vi "Data Save Edit.vi"(10 "Data Path":path, 11 "Project":string) -> (3 "OK?":bool)   [LabVIEW 2020]
uses:
  <vilib>/Utility/miscctls.llb/LVMapReplaceAction.ctl
  <vilib>/Utility/file.llb/Write Delimited Spreadsheet (string).vi
  <vilib>/Utility/config.llb/Read Key (String).vi
  <vilib>/Utility/file.llb/Read Delimited Spreadsheet (string).vi
  <vilib>/Utility/config.llb/NI_LVConfig.lvlib
panel:
  in  "Warning Group Delete":bool
  in  "Warning Group Add":bool
  in  "WarningGroup":i32(listbox)
  in  "Warning Delete":bool
  in  "Warning Export":bool
  in  "Warning Import":bool
  in  "Warning Edit":bool
  in  "Warning List":i32(listbox) caption="报警日志"
  in  "OK":bool
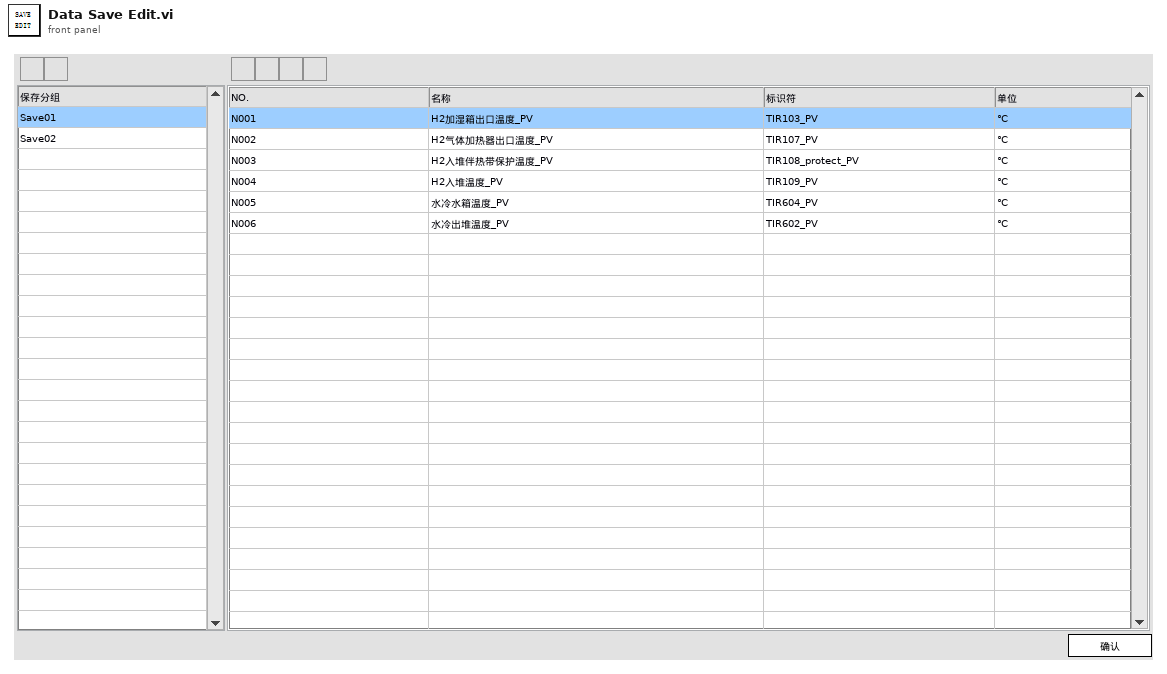
[diagram p1: front panel]
types:
  T1 = cluster{"Project":string, "Warning List":string[][], "OK?":bool, "Warning":map{string, cluster{"Name":string, "ID":string, "Unit":string}}, "Data Path":path, "Warning0":refnum<vi>, "WarningContent":refnum<vi>, "Formular List0":string[], "Value":i32}
  T2 = typedef "LVMapReplaceAction.ctl" = enum32{"Modify Entry only if found", "Add or Modify Entry", "Delete Entry"}
  T3 = typedef "NI_LVConfig.lvlib/Config Data RefNum.ctl" = refnum<k1>
  T4 = map{string, cluster{"Name":string, "ID":string, "Unit":string}}
  T5 = cluster{"Name":string, "ID":string, "Unit":string}
  T6 = typedef "SDQ Data Type.ctl" = cluster{"CAN Length":string, "CAN Name":string, "CAN ID":string, "CAN Type":string, "Test Item":string, "Byte Order":string, "Instruction":string, "Control Type":string, "Group":string, "Offset":dbl, "Coefficient":dbl, "Write Enable":bool, "Lable Type":string, "Key?":string, "Set Value":string, "Upper":dbl, "Lower":dbl, "Unit":string, "Formula":string, "Test Item Type":string, "Length":i32, "Address":string, "Name":string, "Identifier":string, "Data Type":string, "Enumerate?":string, "Enumerate List":string, "Data":string, "Source":string}
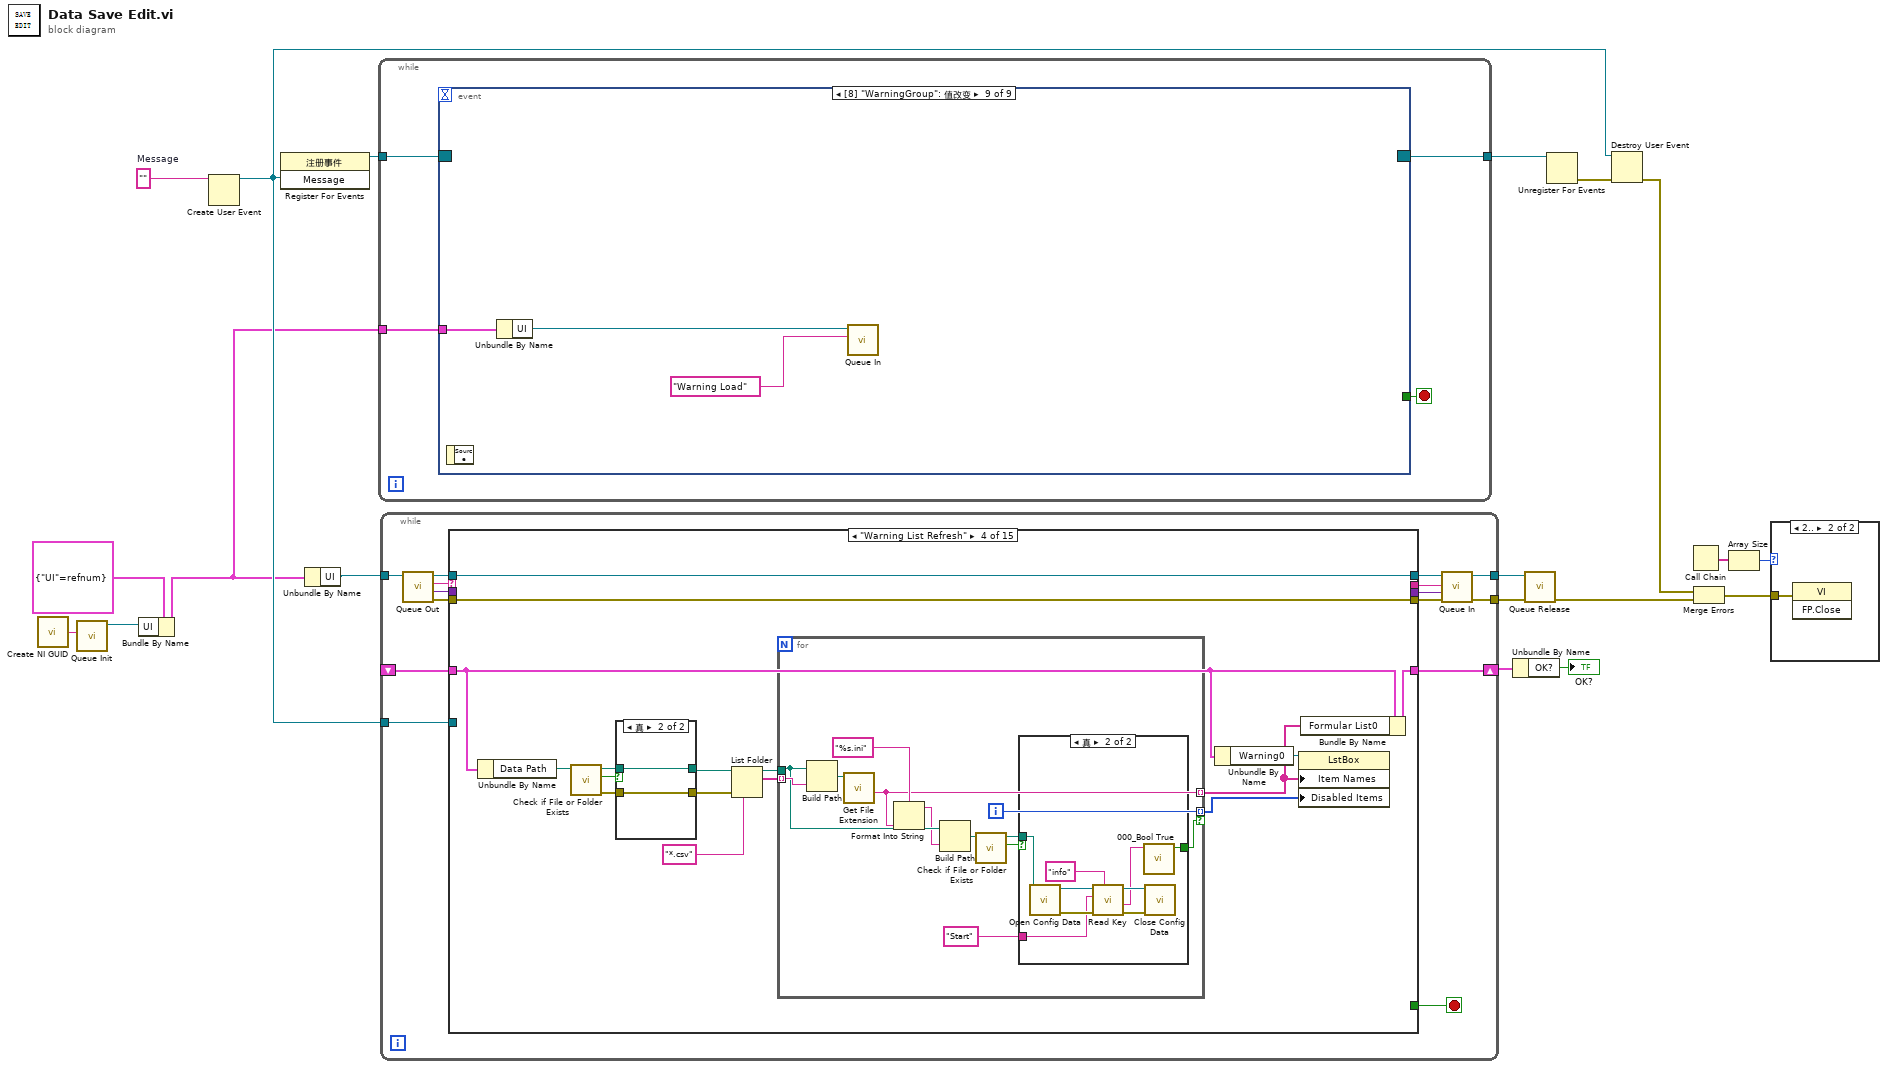
[diagram p0: block diagram]
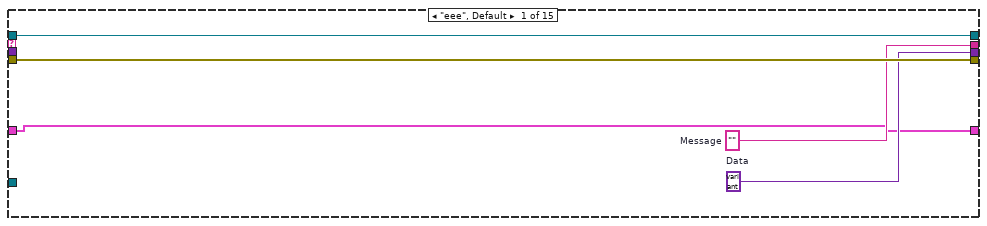
[diagram p3: hidden frame]
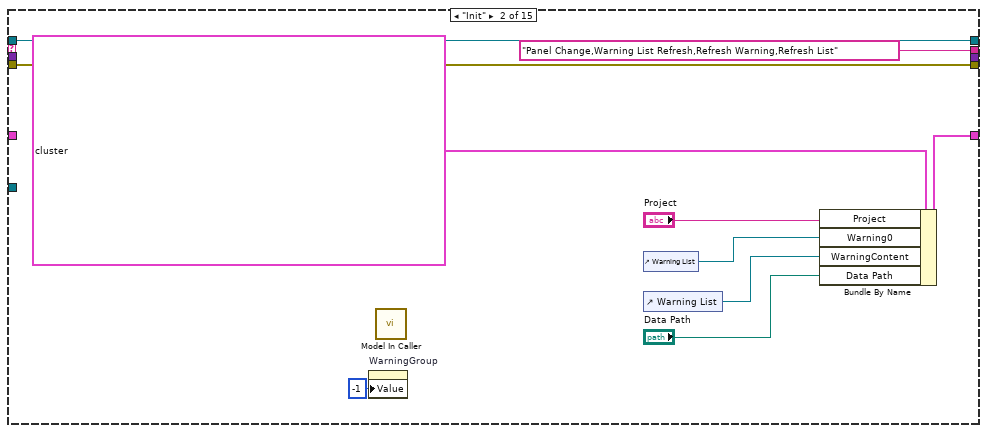
[diagram p4: hidden frame]
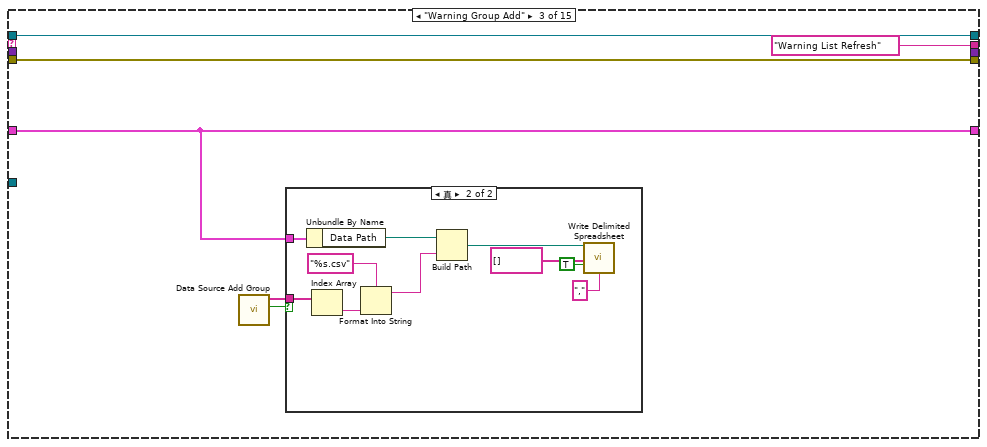
[diagram p5: hidden frame]
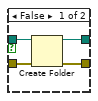
[diagram p8: hidden frame]
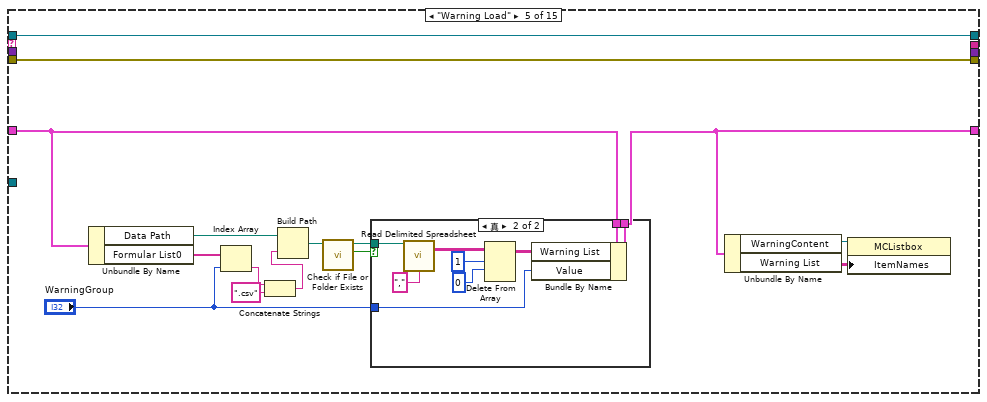
[diagram p9: hidden frame]
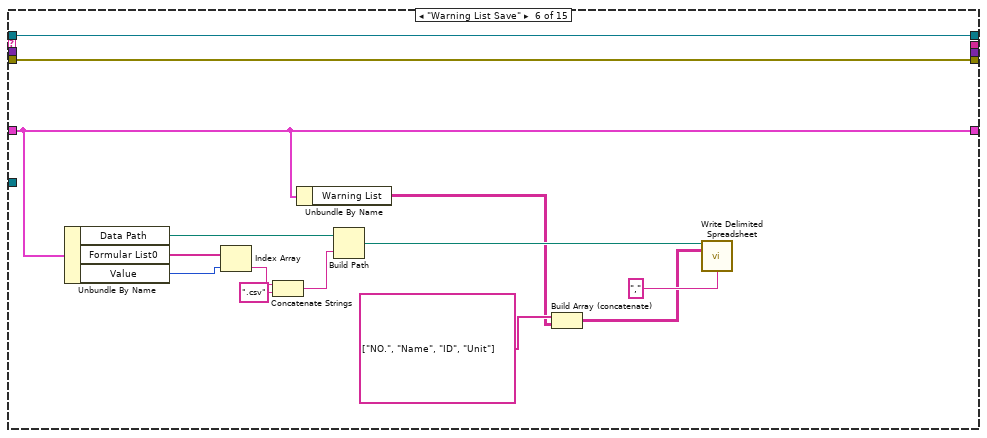
[diagram p11: hidden frame]
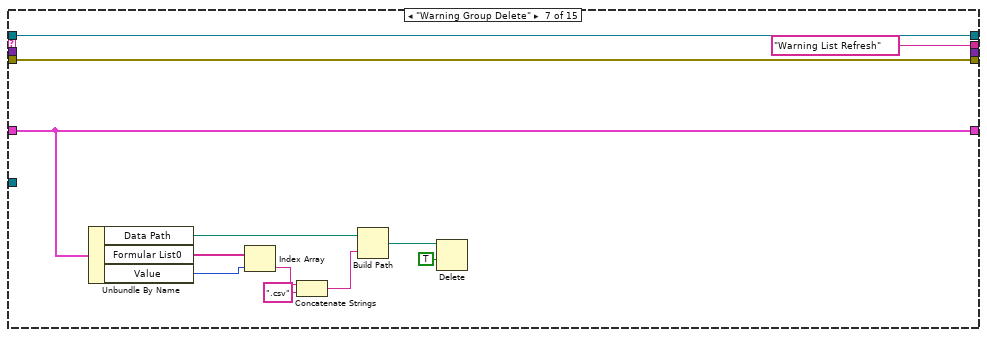
[diagram p12: hidden frame]
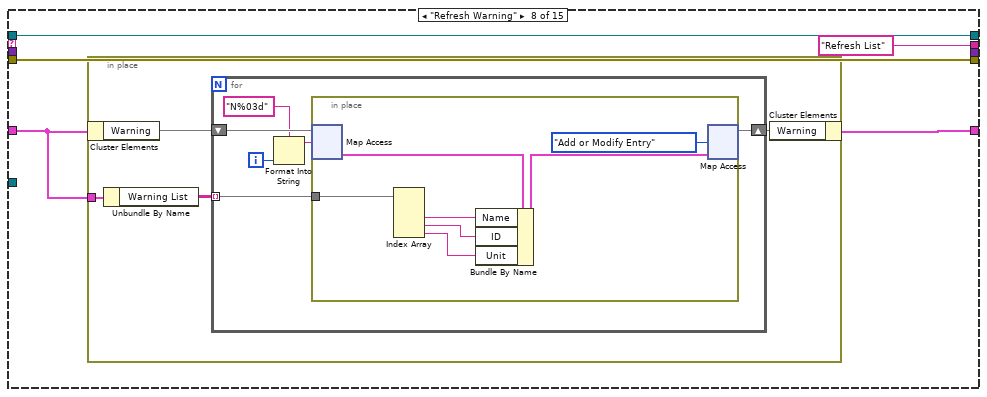
[diagram p13: hidden frame]
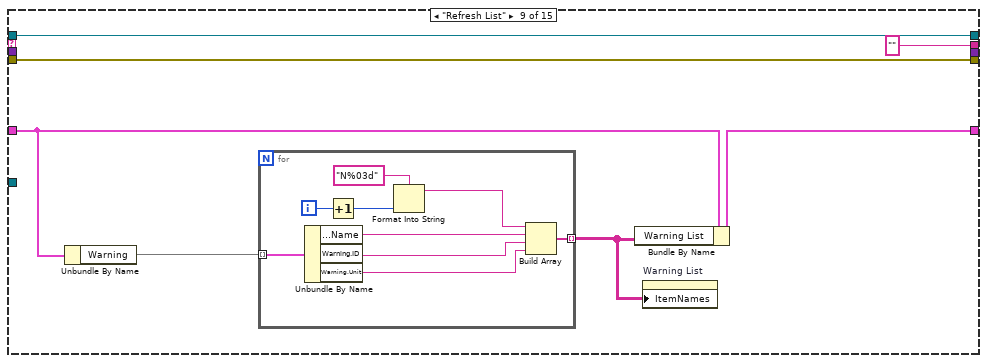
[diagram p14: hidden frame]
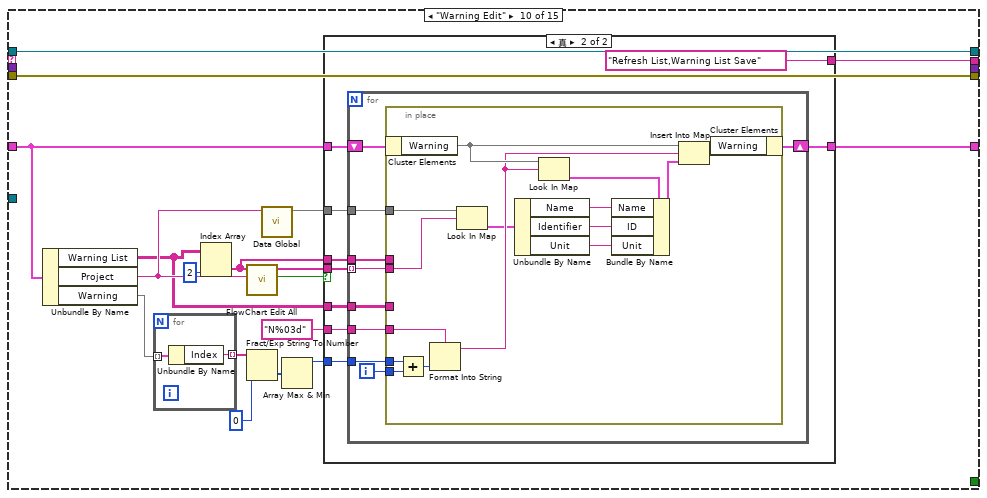
[diagram p15: hidden frame]
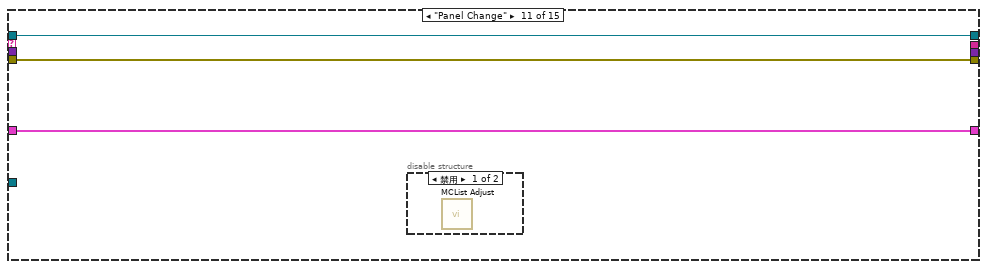
[diagram p17: hidden frame]
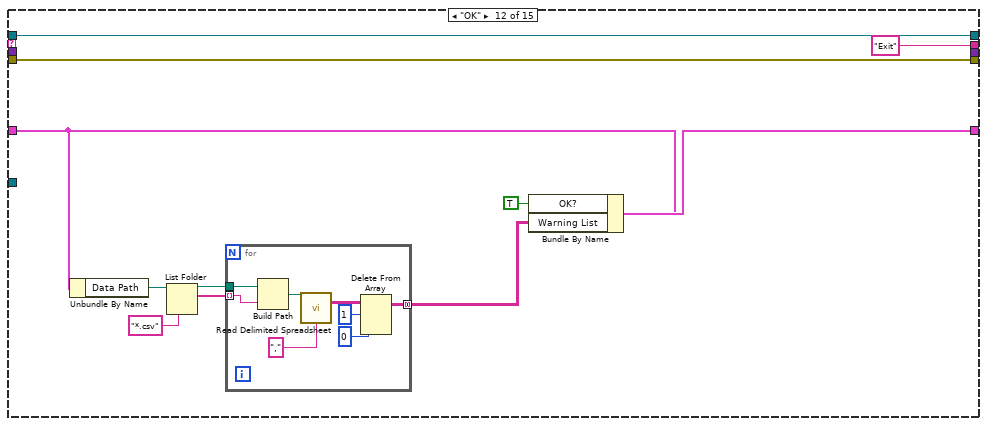
[diagram p19: hidden frame]
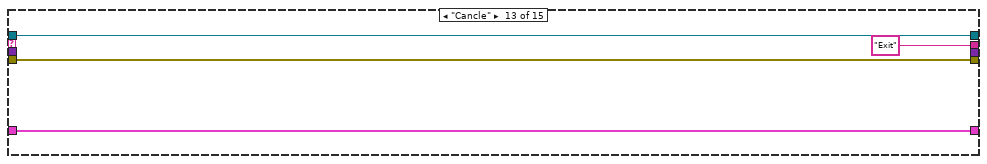
[diagram p20: hidden frame]
diagram:
  w7 = ""  # Message
  n1 = call <vilib>:"Create NI GUID.vi"() -> ("NI GUID"=w5:string)
  n2 = call "Queue Init.vi"("Queue Name"=w5) -> ("Queue Out"=w3:refnum<queue>)  [unwired: 8 in, 2 out]
  n3 = Bundle By Name(cluster=cluster{"UI":refnum<queue>} {"UI"=refnum} ("Queue Ref Out"), "UI"=w3) -> (w4:cluster{"UI":refnum<queue>})
  n4 = Create User Event(user event datatype=w7) -> (user event=w11:refnum<user-event>)  [unwired: 1 in, 1 out]
  n5 = register-events(w11) -> (reference out=w8:refnum<event-registration>)  [unwired: 2 in, 1 out]
  n6 = Unbundle By Name(w4) -> ("UI"=w14:refnum<queue>)
  n7 = while {
    tunnel: w8 -> [w23]
    tunnel: [w21] -> w9
    tunnel: w4 -> [w20]
    stop <- w22 stop-if-true
    n8 = event shown="[8] \"WarningGroup\": 值改变" {
      selector: w23 -> [_ _ _ _ _ _ _ _ _]
      dyn-events: [_ _ _ _ _ _ _ _ _] -> w21
      timeout: _ -> [_ _ _ _ _ _ _ _ _]
      tunnel: [_ _ _ _ w35 _ _ _ _] -> w22
      tunnel: w20 -> [_ _ w30 w33 _ w40 w45 w48 w51]
      event Timeout {
        n9 = event-data() -> ()  [unwired: 1 in, 1 out]
      }
      event Key Down {
        n10 = event-data() -> ("Char"=w25:i16, "PlatMods.Ctrl"=w24:bool)  [unwired: 1 in]
        n11 = case shown="真" w24 {
          tunnel: w25 -> [_ w26]
          frame False {
          }
          frame True {
            n12 = case shown="101" w26 {
              frame 0, Default {
              }
              frame 101 {
                n13 = property class="VI"("BDWin.Open"=TRUE ("程序框图窗口:打开")) -> ()  [unwired: 2 in, 2 out]
              }
            }
          }
        }
      }
      event Panel Resize {
        n14 = event-data() -> ()  [unwired: 1 in, 1 out]
        n15 = Unbundle By Name(w30) -> ("UI"=w29:refnum<queue>)
        n16 = call "Queue In.vi"("Message"="Panel Change", "Queue In"=w29) -> ()  [unwired: 8 in, 2 out]
      }
      event "OK": Value Change {
        n17 = event-data() -> ("CtlRef"=w34:refnum<vi>)  [unwired: 1 in]
        n18 = property class="Bool"(reference=w34) -> ("Label.Text"=w31:string)  [unwired: 1 in, 2 out]
        n19 = Unbundle By Name(w33) -> ("UI"=w32:refnum<queue>)
        n20 = call "Queue In.vi"("Message"=w31, "Queue In"=w32) -> ()  [unwired: 8 in, 2 out]
      }
      event User Event {
        n21 = event-data() -> ("Message"=w37:string)  [unwired: 1 in]
        n22 = Equal?(x=w37, y="Exit") -> (x = y?=w35:bool)
      }
      event Panel Close? {
        n23 = event-data() -> ()  [unwired: 1 in, 1 out]
        n24 = Unbundle By Name(w40) -> ("UI"=w39:refnum<queue>)
        n25 = call "Queue In.vi"("Message"="Exit", "Queue In"=w39) -> ()  [unwired: 8 in, 2 out]
        n26 = event-data("Discard?"=TRUE ("放弃？")) -> ()  [unwired: 1 in, 1 out]
      }
      event "Warning Edit", "Warning Import", "Warning Export", "Warning Delete", "Warning Group Add", "Warning Group Delete": Value Change {
        n27 = event-data() -> ("CtlRef"=w44:refnum<vi>)  [unwired: 1 in]
        n28 = Unbundle By Name(w45) -> ("UI"=w43:refnum<queue>)
        n29 = property class="Bool"(reference=w44) -> ("Label.Text"=w42:string)  [unwired: 1 in, 2 out]
        n30 = call "Queue In.vi"("Message"=w42, "Queue In"=w43) -> ()  [unwired: 8 in, 2 out]
      }
      event "Warning List": Double Click {
        n31 = event-data() -> ()  [unwired: 1 in, 1 out]
        n32 = Unbundle By Name(w48) -> ("UI"=w47:refnum<queue>)
        n33 = call "Queue In.vi"("Message"="Warning Edit", "Queue In"=w47) -> ()  [unwired: 8 in, 2 out]
      }
      event "WarningGroup": Value Change {
        n34 = event-data() -> ()  [unwired: 1 in, 1 out]
        n35 = Unbundle By Name(w51) -> ("UI"=w50:refnum<queue>)
        n36 = call "Queue In.vi"("Message"="Warning Load", "Queue In"=w50) -> ()  [unwired: 8 in, 2 out]
      }
    }
  }
  n37 = while {
    tunnel: w14 -> [w61]
    tunnel: [w58] -> w12
    tunnel: [w57] -> w13
    tunnel: w11 -> [w65]
    shift-right: [w53] -> w2
    shift-left: _ -> [w52]
    stop <- w66 stop-if-true
    n38 = call "Queue Out.vi"("Queue In"=w61) -> ("error out"=w64:errorcluster, "Data"=w62:variant, "Message"=w63:string, "Queue Out"=w60:refnum<queue>)  [unwired: 6 in, 1 out]
    n39 = case shown="\"Warning List Refresh\"" w63 {
      selector: w63 -> [_ _ _ _ _ _ _ _ _ _ _ _ _ w311 _]
      tunnel: w60 -> [w71 w81 w87 w113 w155 w179 w191 w196 w220 w247 w286 w297 w309 w315 w320]
      tunnel: w64 -> [w70 w80 w86 w112 w154 w178 w190 w195 w219 w246 w285 w296 w308 w313 w321]
      tunnel: [w71 w81 w87 w113 w155 w179 w191 w196 w220 w247 w286 w297 w309 w314 w320] -> w59
      tunnel: [w70 w80 w86 w112 w154 w178 w190 w195 w219 w246 w285 w296 w308 w312 w321] -> w56
      tunnel: [w69 "Panel Change,Warning List Refresh,Refresh Warning,Refresh List" ("Message") "Warning List Refresh" ("Message") _ _ _ "Warning List Refresh" ("Message") "Refresh List" ("Message") "" ("Message") w235 _ "Exit" ("Message") "Exit" ("Message") "Quit" _] -> w55
      tunnel: [_ _ _ _ _ _ _ _ _ _ _ _ _ _ TRUE] -> w66
      tunnel: w65 -> [_ _ _ _ _ _ _ _ _ _ _ _ _ w317 _]
      tunnel: [w68 _ _ _ _ _ _ _ _ _ _ _ _ _ _] -> w54
      tunnel: w62 -> [_ _ _ _ _ _ _ _ _ _ _ _ _ _ _]
      tunnel: [w67 w77 w83 w102 w141 w172 w184 w194 w216 w241 w284 w294 w306 w310 w318] -> w53
      tunnel: w52 -> [w67 _ w83 w103 w143 w172 w184 w193 w218 w242 w284 w292 w306 w310 w318]
      frame "eee", Default {
        w68 = variant  # Data
        w69 = ""  # Message
      }
      frame "Init" {
        n40 = property on="WarningGroup" class="LstBox (严格)"("Value"=-1 ("WarningGroup")) -> ()  [unwired: 2 in, 2 out]
        n41 = call "Model In Caller.vi"() -> ()  [unwired: 11 in, 1 out]
        n42 = control-ref of="Warning List"() -> (w75:refnum<vi>)
        n43 = control-ref of="Warning List"() -> (w74:refnum<vi>)
        n44 = Bundle By Name(cluster=T1 {"Project"="", "Warning List"=[], "OK?"=FALSE, "Warning"={}, "Data Path"=path "", "Warning0"=refnum, "WarningContent"=refnum, "Formular List0"=[], "Value"=0}, "Project"="Project", "Warning0"=w75, "WarningContent"=w74, "Data Path"="Data Path") -> (w77:T1)
      }
      frame "Warning Group Add" {
        n45 = call "Data Source Add Group.vi"() -> ("OK？"=w85:bool, "Data Out"=w84:string[])  [unwired: 9 in, 1 out]
        n46 = case shown="真" w85 {
          tunnel: w84 -> [_ w97]
          tunnel: w83 -> [_ w96]
          frame False {
          }
          frame True {
            n47 = Unbundle By Name(w96) -> ("Data Path"=w95:path)
            n48 = Index Array(array=w97) -> (element=w93:string)  [unwired: 1 in]
            n49 = Format Into String(format string="%s.csv" ("格式字符串"), w93) -> (resulting string=w92:string)  [unwired: 2 in, 1 out]
            n50 = Build Path(base path=w95, name or relative path=w92) -> (appended path=w91:path)
            n51 = call-poly <vilib>:"Write Delimited Spreadsheet.vi"("file path (dialog if empty)"=w91, "1D data"=string[] [], "append to file? (new file:F)"=TRUE, "delimiter (\\t)"="," ("delimiter (\\t)")) -> ()  [unwired: 10 in, 2 out]
          }
        }
      }
      frame "Warning List Refresh" {
        n52 = Unbundle By Name(w103) -> ("Data Path"=w104:path)
        n53 = call <vilib>:"Check if File or Folder Exists.vi"("path"=w104) -> ("error out"=w107:errorcluster, "file or folder exists?"=w105:bool, "dup path"=w106:path)  [unwired: 8 in]
        n54 = case shown="真" w105 {
          tunnel: w106 -> [w138 w140]
          tunnel: w107 -> [w137 w139]
          tunnel: [w135 w140] -> w108
          tunnel: [w136 w139] -> w109
          frame False {
            n55 = Create Folder(path (use dialog)=w138, error in=w137) -> (created path=w135:path, error out=w136:errorcluster)  [unwired: 1 in, 1 out]
          }
          frame True {
          }
        }
        n56 = List Folder(path=w108, pattern="*.csv" ("类型"), error in=w109) -> (path out=w100:path, filenames=w101:string[])  [unwired: 1 in, 2 out]
        n57 = for {
          tunnel: w101 -> [w125] mode=indexing
          tunnel: w100 -> [w121]
          tunnel: [w122] -> w99 mode=indexing
          tunnel: [w115] -> w98 mode=indexing if=w114
          i -> [w115]
          n58 = Build Path(base path=w121, name or relative path=w125) -> (appended path=w124:path)
          n59 = call <vilib>:"Get File Extension.vi"("file"=w124) -> ("filename without extension"=w122:string)  [unwired: 6 in, 4 out]
          n60 = Format Into String(format string="%s.ini" ("格式字符串"), w122) -> (resulting string=w120:string)  [unwired: 2 in, 1 out]
          n61 = Build Path(base path=w121, name or relative path=w120) -> (appended path=w119:path)
          n62 = call <vilib>:"Check if File or Folder Exists.vi"("path"=w119) -> ("file or folder exists?"=w117:bool, "dup path"=w116:path)  [unwired: 8 in, 1 out]
          n63 = case shown="真" w117 {
            tunnel: "Start" ("key") -> [_ w128]
            tunnel: w116 -> [_ w127]
            tunnel: [_ w126] -> w114
            frame False {
            }
            frame True {
              n64 = call <vilib>:"Open Config Data.vi"("configuration file path"=w127) -> ("error out"=w133:errorcluster, "refnum"=w134:T3)  [unwired: 8 in, 1 out]
              n65 = call-poly <vilib>:"Read Key.vi"("section"="info", "error in (no error)"=w133, "key"=w128, "refnum"=w134) -> ("error out"=w132:errorcluster, "value"=w129:string, "refnum out"=w131:T3)  [unwired: 4 in, 1 out]
              n66 = call "000_Bool True.vi"("Bool String"=w129) -> ("True"=w126:bool)  [unwired: 8 in, 2 out]
              n67 = call <vilib>:"Close Config Data.vi"("error in (no error)"=w132, "refnum"=w131) -> ()  [unwired: 8 in, 2 out]
            }
          }
        }
        n68 = Unbundle By Name(w103) -> ("Warning0"=w110:refnum<vi>)
        n69 = property class="LstBox"(reference=w110, "Item Names"=w99, "Disabled Items"=w98) -> ()  [unwired: 1 in, 2 out]
        n70 = Bundle By Name(cluster=w103, "Formular List0"=w99) -> (w102:T1)
      }
      frame "Warning Load" {
        n71 = Unbundle By Name(w143) -> ("Data Path"=w144:path, "Formular List0"=w150:string[])
        n72 = Index Array(array=w150, index="WarningGroup") -> (element=w151:string)
        n73 = Concatenate Strings(w151, ".csv" ("字符串")) -> (w153:string)
        n74 = Build Path(base path=w144, name or relative path=w153) -> (appended path=w147:path)
        n75 = call <vilib>:"Check if File or Folder Exists.vi"("path"=w147) -> ("file or folder exists?"=w148:bool, "dup path"=w149:path)  [unwired: 8 in, 1 out]
        n76 = case shown="真" w148 {
          tunnel: w143 -> [w156 w165]
          tunnel: [w156 w159] -> w141
          tunnel: "WarningGroup" -> [_ w158]
          tunnel: w149 -> [_ w157]
          frame False {
          }
          frame True {
            n77 = call-poly <vilib>:"Read Delimited Spreadsheet.vi"("file path (dialog if empty)"=w157, "delimiter (\\t)"="," ("delimiter (\\t)")) -> ("all rows"=w160:string[][])  [unwired: 8 in, 5 out]
            n78 = Delete From Array(array=w160, length=1 ("长度"), index (row)=0 ("索引 (行)")) -> (array with subset deleted=w163:string[][])  [unwired: 1 in, 1 out]
            n79 = Bundle By Name(cluster=w165, "Warning List"=w163, "Value"=w158) -> (w159:T1)
          }
        }
        n80 = Unbundle By Name(w141) -> ("WarningContent"=w146:refnum<vi>, "Warning List"=w145:string[][])
        n81 = property on="属性节点" class="MCListbox"(reference=w146, "ItemNames"=w145) -> ()  [unwired: 1 in, 2 out]
      }
      frame "Warning List Save" {
        n82 = Unbundle By Name(w172) -> ("Data Path"=w173:path, "Formular List0"=w174:string[], "Value"=w171:i32)
        n83 = Index Array(array=w174, index=w171) -> (element=w175:string)
        n84 = Concatenate Strings(w175, ".csv" ("字符串")) -> (w177:string)
        n85 = Unbundle By Name(w172) -> ("Warning List"=w167:string[][])
        n86 = Build Path(base path=w173, name or relative path=w177) -> (appended path=w169:path)
        n87 = Build Array (concatenate)(string[] ["NO.", "Name", "ID", "Unit"], w167) -> (w166:string[][])
        n88 = call-poly <vilib>:"Write Delimited Spreadsheet.vi"("file path (dialog if empty)"=w169, "2D data"=w166, "delimiter (\\t)"="," ("delimiter (\\t)")) -> ()  [unwired: 11 in, 2 out]
      }
      frame "Warning Group Delete" {
        n89 = Unbundle By Name(w184) -> ("Data Path"=w185:path, "Formular List0"=w186:string[], "Value"=w183:i32)
        n90 = Index Array(array=w186, index=w183) -> (element=w187:string)
        n91 = Concatenate Strings(w187, ".csv" ("字符串")) -> (w189:string)
        n92 = Build Path(base path=w185, name or relative path=w189) -> (appended path=w182:path)
        n93 = Delete(path (use dialog)=w182, confirm (F)=TRUE ("确认(F)")) -> ()  [unwired: 3 in, 3 out]
      }
      frame "Refresh Warning" {
        n94 = in-place {
          in-place-border: w193 -> [w200]
          n95 = in-place-cluster #1(w193) -> ("Warning"=w198:T4)
          n96 = Unbundle By Name(w200) -> ("Warning List"=w199:string[][])
          n97 = for {
            tunnel: w199 -> [w201] mode=indexing
            shift-right: [w205] -> w197
            shift-left: w198 -> [w206]
            i -> [w203]
            n98 = Format Into String(format string="N%03d" ("格式字符串"), w203) -> (resulting string=w202:string)  [unwired: 2 in, 1 out]
            n99 = in-place {
              in-place-border: w201 -> [w210]
              n100 = in-place-map #2(w206, w202) -> (w213:T5)  [unwired: 1 in, 1 out]
              n101 = Index Array(array=w210) -> (element #2=w209:string, element #3=w208:string, element #4=w207:string)  [unwired: 4 in, 1 out]
              n102 = Bundle By Name(cluster=w213, "Name"=w209, "ID"=w208, "Unit"=w207) -> (w211:T5)
              n103 = in-place-map #2(w211, LVMapReplaceAction."Add or Modify Entry" ("操作")) -> (w205:T4)  [unwired: 2 out]
            }
          }
          n104 = in-place-cluster #1("Warning"=w197) -> (w194:T1)
        }
      }
      frame "Refresh List" {
        n105 = Unbundle By Name(w218) -> ("Warning"=w217:T4)
        n106 = for {
          tunnel: w217 -> [w229] mode=indexing
          tunnel: [w227] -> w215 mode=indexing
          i -> [w225]
          n107 = Unbundle By Name(w229) -> ("Warning.Name"=w222:string, "Warning.ID"=w228:string, "Warning.Unit"=w221:string)
          n108 = Increment(x=w225) -> (x+1=w224:i32)
          n109 = Format Into String(format string="N%03d" ("格式字符串"), w224) -> (resulting string=w223:string)  [unwired: 2 in, 1 out]
          n110 = Build Array(w223, w222, w228, w221) -> (w227:string[])
        }
        n111 = Bundle By Name(cluster=w218, "Warning List"=w215) -> (w216:T1)
        n112 = property on="Warning List" class="MCListbox (严格)"("ItemNames"=w215) -> ()  [unwired: 2 in, 2 out]
      }
      frame "Warning Edit" {
        n113 = Unbundle By Name(w242) -> ("Warning List"=w231:string[][], "Project"=w234:string, "Warning"=w240:T4)
        n114 = for {
          tunnel: w240 -> [w249] mode=indexing
          tunnel: [w248] -> w239 mode=indexing
          n115 = Unbundle By Name(w249) -> ("Index"=w248:string)
        }
        n116 = Index Array(array=w231, index (col)=2 ("禁用的索引 (列)")) -> (element=w232:string[])  [unwired: 1 in]
        n117 = call "FlowChart Edit All.vi"("Name"=w234, "Identifier In"=w232) -> ("OK？"=w245:bool, "Identifiers Out"=w244:string[])  [unwired: 8 in]
        n118 = Fract/Exp String To Number(string=w239, default (0 dbl)=0 ("默认(0 DBL)")) -> (number=w238:i32[])  [unwired: 2 in, 1 out]
        n119 = call "Data Global.vi"("Name"=w234) -> ("Data Out"=w233:map{string, T6})  [unwired: 7 in, 3 out]
        n120 = Array Max & Min(array=w238) -> (max value=w237:i32)  [unwired: 3 out]
        n121 = case shown="真" w245 {
          tunnel: w244 -> [_ w257]
          tunnel: w242 -> [w250 w259]
          tunnel: [w250 w258] -> w241
          tunnel: w237 -> [_ w256]
          tunnel: [_ "Refresh List,Warning List Save"] -> w235
          tunnel: w233 -> [_ w254]
          tunnel: w232 -> [_ w253]
          tunnel: w231 -> [_ w252]
          tunnel: "N%03d" ("格式字符串") -> [_ w251]
          frame False {
          }
          frame True {
            n122 = for {
              tunnel: w257 -> [w266] mode=indexing
              tunnel: w256 -> [w265]
              shift-right: [w267] -> w258
              shift-left: w259 -> [w268]
              tunnel: w254 -> [w263]
              tunnel: w253 -> [w262]
              tunnel: w252 -> [w261]
              tunnel: w251 -> [w260]
              i -> [w264]
              n123 = in-place {
                in-place-border: w266 -> [w271]
                in-place-border: w265 -> [w279]
                in-place-border: w264 -> [w277]
                in-place-border: w263 -> [w275]
                in-place-border: w262 -> [_]
                in-place-border: w261 -> [_]
                in-place-border: w260 -> [w270]
                n124 = in-place-cluster #3(w268) -> ("Warning"=w283:T4)
                n125 = Add(x=w279, y=w277) -> (x+y=w278:i32)
                n126 = Format Into String(format string=w270, w278) -> (resulting string=w276:string)  [unwired: 2 in, 1 out]
                n127 = Look In Map(map=w275, key=w271) -> (value=w274:T6)  [unwired: 1 in, 1 out]
                n128 = Unbundle By Name(w274) -> ("Name"=w273:string, "Identifier"=w272:string, "Unit"=w269:string)
                n129 = Look In Map(map=w283, key=w276) -> (value=w281:T5)  [unwired: 1 in, 1 out]
                n130 = Bundle By Name(cluster=w281, "Name"=w273, "ID"=w272, "Unit"=w269) -> (w280:T5)
                n131 = Insert Into Map(map in=w283, key=w276, value=w280) -> (map out=w282:T4)  [unwired: 2 out]
                n132 = in-place-cluster #3("Warning"=w282) -> (w267:T1)
              }
            }
          }
        }
      }
      frame "Panel Change" {
        n133 = disable-structure shown="禁用" {
          frame Disabled {
            n134 = call "MCList Adjust.vi"() -> ()  [unwired: 11 in, 1 out]
          }
          frame Enabled {
          }
        }
      }
      frame "OK" {
        n135 = Unbundle By Name(w292) -> ("Data Path"=w291:path)
        n136 = List Folder(path=w291, pattern="*.csv" ("类型")) -> (path out=w289:path, filenames=w290:string[])  [unwired: 2 in, 2 out]
        n137 = for {
          tunnel: w290 -> [w304] mode=indexing
          tunnel: w289 -> [w305]
          tunnel: [w298] -> w288 mode=concatenating
          n138 = Build Path(base path=w305, name or relative path=w304) -> (appended path=w303:path)
          n139 = call-poly <vilib>:"Read Delimited Spreadsheet.vi"("file path (dialog if empty)"=w303, "delimiter (\\t)"="," ("delimiter (\\t)")) -> ("all rows"=w301:string[][])  [unwired: 8 in, 5 out]
          n140 = Delete From Array(array=w301, length=1 ("长度"), index (row)=0 ("索引 (行)")) -> (array with subset deleted=w298:string[][])  [unwired: 1 in, 1 out]
        }
        n141 = Bundle By Name(cluster=w292, "OK?"=TRUE, "Warning List"=w288) -> (w294:T1)
      }
      frame "Cancle" {
      }
      frame "Exit" {
        n142 = Generate User Event(user event=w317, event data cluster=w311) -> ()  [unwired: 2 in, 2 out]
        n143 = call "Queue Clear.vi"("error in (no error)"=w313, "Queue In"=w315) -> ("error out"=w312:errorcluster, "Queue Out"=w314:refnum<queue>)  [unwired: 8 in]
      }
      frame "Quit" {
      }
    }
    n144 = call "Queue In.vi"("error in (no error)"=w56, "Data"=w54, "Message"=w55, "Queue In"=w59) -> ("error out"=w57:errorcluster, "Queue Out"=w58:refnum<queue>)  [unwired: 6 in]
  }
  n145 = Unbundle By Name(w2) -> ("OK?"=→"OK?":bool)
  n146 = call "Queue Release.vi"("error in (no error)"=w13, "Queue In"=w12) -> ("error out"=w16:errorcluster)  [unwired: 9 in]
  n147 = Unregister For Events(event registration refnum=w9) -> (error out=w10:errorcluster)  [unwired: 1 in]
  n148 = Destroy User Event(user event=w11, error in=w10) -> (error out=w15:errorcluster)
  n149 = Call Chain() -> (call chain=w18:string[])
  n150 = Merge Errors(w15, w16) -> (w17:errorcluster)
  n151 = Array Size(array=w18) -> (size(s)=w19:i32)
  n152 = case shown="2.." w19 {
    tunnel: w17 -> [_ w322]
    frame 0, Default {
    }
    frame 2.. {
      n153 = invoke class="VI" method="FP.Close"(error in=w322) -> ()  [unwired: 2 in, 3 out]
    }
  }
